vi "Camera Status.vi"(11 "Digital input":bool[](array[boolean])) -> (2 "Camera Status":T1)   [LabVIEW 2015]
panel:
  in  "Cluster":T1
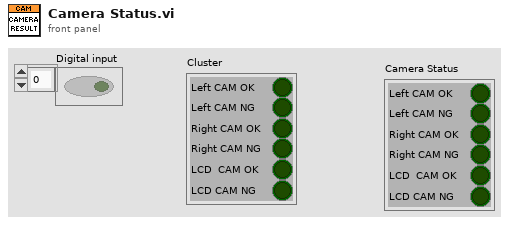
[diagram p1: front panel]
types:
  T1 = cluster{"Left CAM OK":bool, "Left CAM NG":bool, "Right CAM OK":bool, "Right CAM NG":bool, "LCD  CAM OK":bool, "LCD CAM NG ":bool}
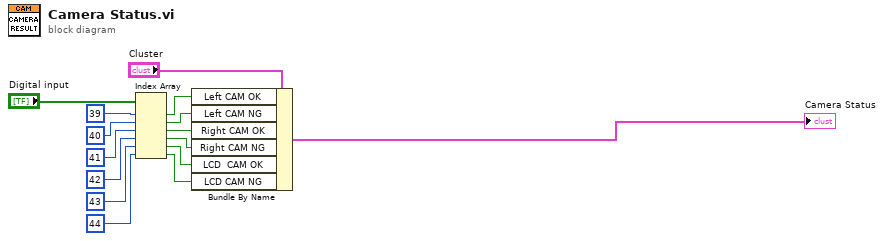
[diagram p0: block diagram]
diagram:
  n1 = Index Array(array="Digital input", index #1=39 ("index"), index #2=40 ("index"), index #3=41 ("index"), index #4=42 ("index"), index #5=43 ("index"), index #6=44 ("index")) -> (element #1=w7:bool, element #2=w6:bool, element #3=w5:bool, element #4=w4:bool, element #5=w3:bool, element #6=w2:bool)
  n2 = Bundle By Name(cluster="Cluster", "Left CAM OK"=w7, "Left CAM NG"=w6, "Right CAM OK"=w5, "Right CAM NG"=w4, "LCD  CAM OK"=w3, "LCD CAM NG"=w2) -> (→"Camera Status":T1)
